vi "Read Units.vi"(8 "error in (no error)":errorcluster, 11 "Floating Point in":refnum<class "Abs_Floating Point.lvclass">) -> (0 "error out":errorcluster, 2 "Units":string, 3 "Floating Point out":refnum<class "Abs_Floating Point.lvclass">)   [LabVIEW 2021, in "Abs_Floating Point.lvclass"]
uses:
  Abs_Floating Point.lvclass
  Abs_Floating Point.lvclass/Abs_Floating Point.ctl
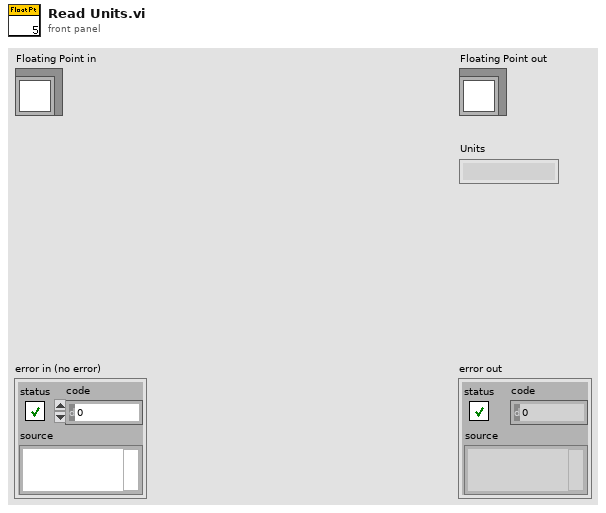
[diagram p1: front panel]
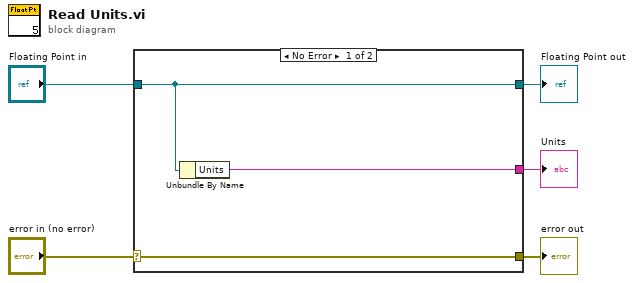
[diagram p0: block diagram]
diagram:
  n1 = case shown="No Error" "error in (no error)" {
    selector: "error in (no error)" -> [w8 w9]
    tunnel: [w8 w9] -> w4
    tunnel: [w7 w10] -> w2
    tunnel: "Floating Point in" -> [w7 w10]
    tunnel: [w6 _] -> w1
    frame No Error {
      n2 = Unbundle By Name(w7) -> ("Units"=w6:string)
    }
    frame Error {
    }
  }
  "error out" <- w4
  "Floating Point out" <- w2
  "Units" <- w1
